vi "Remove_Quotes.vi"(1 "String":string) -> (0 "String Out":string)   [LabVIEW 2010]
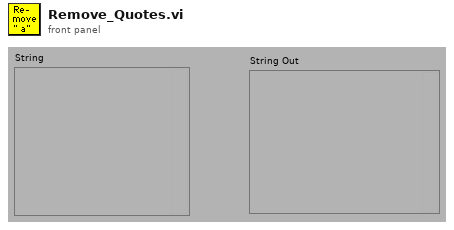
[diagram p1: front panel]
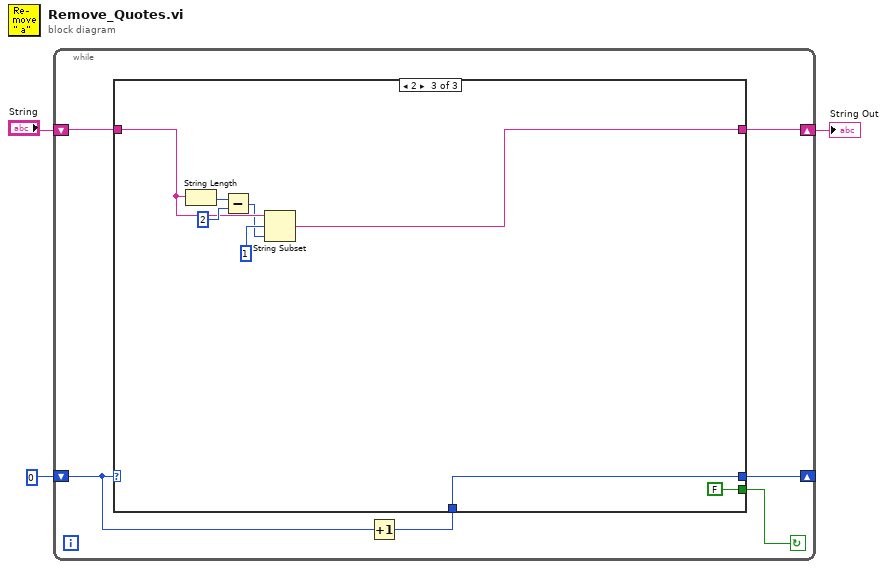
[diagram p0: block diagram]
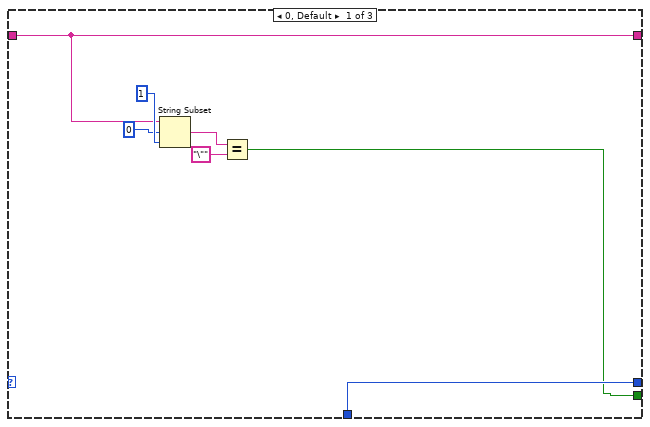
[diagram p2: hidden frame]
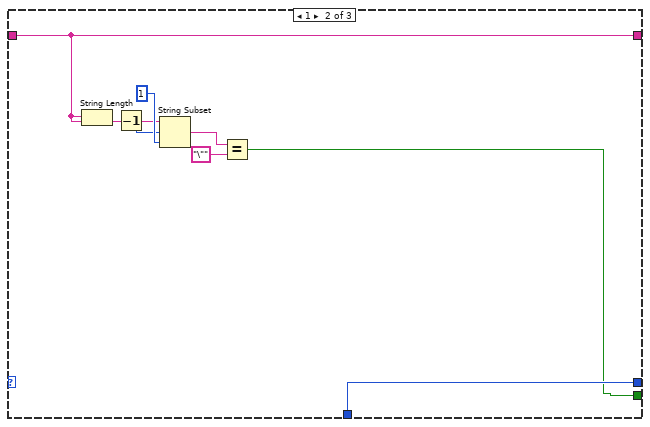
[diagram p3: hidden frame]
diagram:
  n1 = while {
    shift-left: "String" -> [w5]
    shift-right: [w4] -> w1
    shift-left: 0 -> [w8]
    shift-right: [w6] -> _
    stop <- w9 continue-if-true
    n2 = Increment(x=w8) -> (x+1=w7:i32)
    n3 = case shown="2" w8 {
      tunnel: [w10 w20 FALSE] -> w9
      tunnel: w7 -> [w16 w24 w32]
      tunnel: [w16 w24 w32] -> w6
      tunnel: w5 -> [w12 w19 w27]
      tunnel: [w12 w19 w25] -> w4
      frame 0, Default {
        n4 = String Subset(string=w12, offset (0)=0, length (rest)=1 ("length")) -> (substring=w11:string)
        n5 = Equal?(x=w11, y="\"") -> (x = y?=w10:bool)
      }
      frame 1 {
        n6 = String Length(string=w19) -> (length=w18:i32)
        n7 = Decrement(x=w18) -> (x-1=w17:i32)
        n8 = String Subset(string=w19, offset (0)=w17, length (rest)=1 ("length")) -> (substring=w21:string)
        n9 = Equal?(x=w21, y="\"") -> (x = y?=w20:bool)
      }
      frame 2 {
        n10 = String Length(string=w27) -> (length=w29:i32)
        n11 = Subtract(x=w29, y=2) -> (x-y=w26:i32)
        n12 = String Subset(string=w27, offset (0)=1 ("length"), length (rest)=w26) -> (substring=w25:string)
      }
    }
  }
  "String Out" <- w1
